vi "test sv host.vi"() -> ()   [LabVIEW 2012]
panel:
  out "timed out?":bool
  out "ServerStart":bool
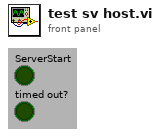
[diagram p1: front panel]
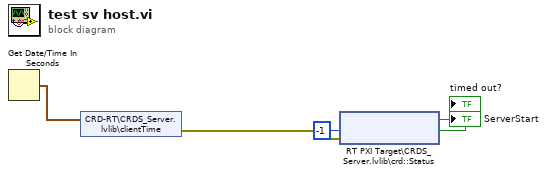
[diagram p0: block diagram]
diagram:
  n1 = Get Date/Time In Seconds() -> (seconds since 1Jan1904=w5:timestamp)
  n2 = shared-variable "CRD-RT\\CRDS_Server.lvlib\\clientTime"(w5) -> (error out=w4:errorcluster)  [unwired: 1 in]
  n3 = shared-variable "RT PXI Target\\CRDS_Server.lvlib\\crd::Status"(error in=w4, -1 ("ms timeout (0)")) -> (→"ServerStart":bool, →"timed out?":bool)  [unwired: 1 out]
